vi "ReadProdModel.vi"(8 "error in":errorcluster caption="错误输入（无错误）", 11 "产品型号":refnum<vi>) -> (0 "error out":errorcluster caption="错误输出")   [LabVIEW 2013]
uses:
  GlobValue.vi
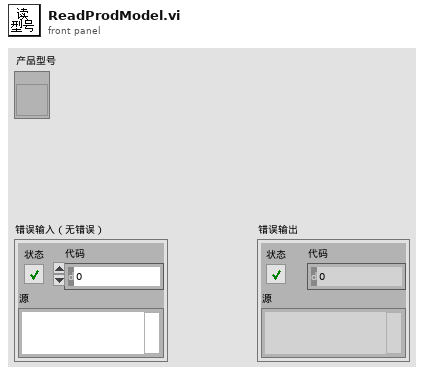
[diagram p1: front panel]
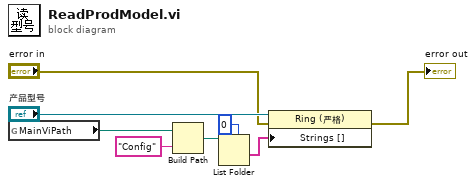
[diagram p0: block diagram]
diagram:
  n1 = global read "GlobValue.vi" "MainViPath"() -> (w1:path)
  n2 = Build Path(base path=w1, name or relative path="Config" ("名称或相对路径")) -> (appended path=w6:path)
  n3 = List Folder(datalog type=0 ("数据记录类型"), path=w6) -> (folder names=w5:string[])  [unwired: 2 in, 3 out]
  n4 = property class="Ring (严格)"(reference="产品型号", error in="error in", "Strings []"=w5) -> (error out=→"error out":errorcluster)  [unwired: 1 out]
